vi "Create.vi"(8 "error in (no error)":errorcluster, 9 "String Buffer (null)":refnum<class "Buffer.lvclass">, 10 "Async Buffer (null)":refnum<class "Buffer.lvclass">, 11 "Inline Buffer (null)":refnum<class "Buffer.lvclass">) -> (0 "error out":errorcluster, 3 "Buffers out":refnum<class "Buffers.lvclass">)   [LabVIEW 2020, in "DSF Core.lvlib" / "Buffers.lvclass"]
uses:
  Buffers.lvclass
  Buffer/Buffer.lvclass
  Buffers.lvclass/Buffers.ctl
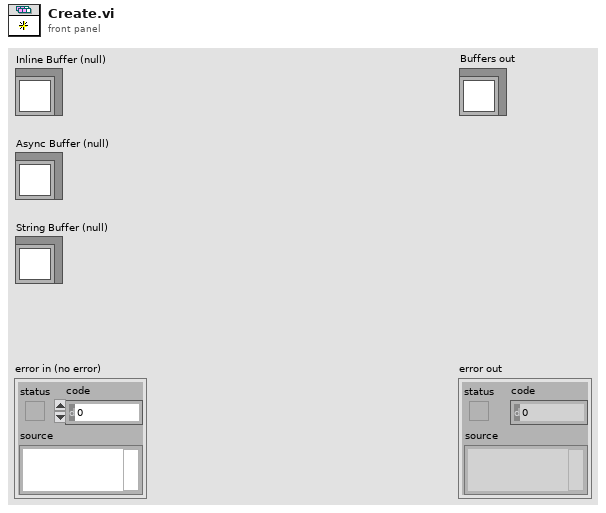
[diagram p1: front panel]
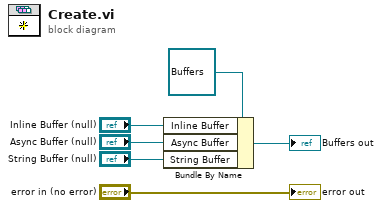
[diagram p0: block diagram]
diagram:
  n1 = Bundle By Name(cluster=refnum<class "Buffers.lvclass"> refnum ("Buffers in"), "Inline Buffer"="Inline Buffer (null)", "Async Buffer"="Async Buffer (null)", "String Buffer"="String Buffer (null)") -> (→"Buffers out":refnum<class "Buffers.lvclass">)
  "error out" <- "error in (no error)"
